vi "CLUSTERSimple.vi"() -> ()   [LabVIEW 2023]
doc: "This function takes a cluster that contains a DBL, I32, and Boolean (in that order) as input. It squares the value of the DBL, halves the value of the I32, and inverts the Boolean. The result is returned in output.\n\nFor information on the data types used for the DLL function, right-click on the Call Library Function node and choose Configure."
uses:
  CLF_Example.dll
panel:
  out "output":cluster{"DBL":dbl, "I32":i32, "Boolean":bool}
  in  "input":cluster{"DBL":dbl, "I32":i32, "Boolean":bool}={"DBL"=10.0, "I32"=5, "Boolean"=FALSE}
  # "See the block diagram for more information."
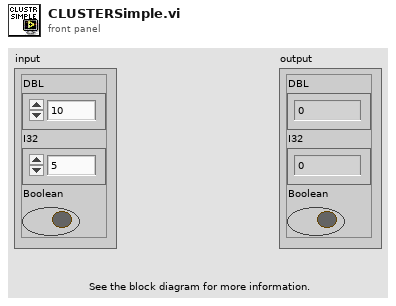
[diagram p1: front panel]
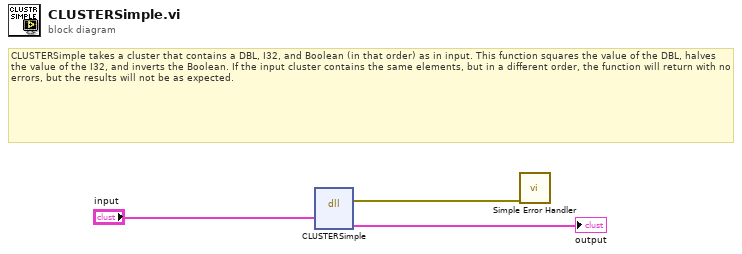
[diagram p0: block diagram]
diagram:
  # "CLUSTERSimple takes a cluster that contains a DBL, I32, and Boolean (in that order) as in input. This function squares the value of the DBL, halves the value of the I32, and inverts the Boolean. If the input cluster contains the same elements, but in a different order, the function will return with no errors, but the results will not be as expected."
  n1 = dll-call lib="c:/dev/_r/4/eng/lv-core/lvpostprocessingd/lv_mc_x86_64/dist_i386/examples/Connectivity/Libraries and Executables/DLL Calling VIs/CLF_Example**.*" fn="CLUSTERSimple"("input"="input") -> (error out=w1:errorcluster, "output"=→"output":cluster{"DBL":dbl, "I32":i32, "Boolean":bool})  [unwired: 4 in, 3 out]
  n2 = call <vilib>:"Simple Error Handler.vi"("error in (no error)"=w1) -> ()  [unwired: 4 in, 5 out]
